vi "Interpolation.vi"() -> (2 "Flywheel Interp":dbl, 3 "Hood Interp":dbl format="%0.2f")   [LabVIEW 2025]
uses:
  <vilib>/Rock Robotics/Network Tables/NT Read Number.vi
  Framework/Robot Global Data.vi
  <vilib>/gmath/NI_Gmath.lvlib
  <vilib>/ptbypt/NI_PtbyPt.lvlib
panel:
  out "Distance to hub":dbl
  in  "Flywheel Long":dbl[](array[numeric])=[0.0, 2000.0, 2000.0, 2500.0, 2500.0, 2500.0, 2500.0, 2500.0, 2500.0, 2500.0, 3000.0, 3000.0, 3500.0, 3500.0]
  in  "Hood Long":dbl[](array[numeric])=[0.0, 40.0, 35.0, 32.0, 30.0, 25.0, 22.0, 19.0, 16.0, 13.0, 10.0, 8.0, 4.5, 2.5]
  in  "Distances Long":dbl[](array[numeric])=[0.0, 63.207, 78.8079, 85.5428, 94.7436, 106.213, 113.25, 133.336, 150.843, 165.063, 172.918, 195.81, 222.008, 256.275]
  in  "Flywheel":dbl[](array[numeric])=[3200.0, 3400.0, 3650.0, 3750.0, 3850.0, 4050.0, 4150.0, 4500.0, 4900.0, 2500.0, 3000.0, 3000.0, 3500.0, 3500.0]
  in  "Hood":dbl[](array[numeric])=[2850.0, 2900.0, 3100.0, 3200.0, 3250.0, 3350.0, 3400.0, 3900.0, 4200.0, 13.0, 10.0, 8.0, 4.5, 2.5]
  in  "Distances":dbl[](array[numeric])=[4.35402, 5.41468, 6.21537, 7.05234, 7.9447, 8.90908, 9.99438, 10.7736, 11.912, 165.063, 172.918, 195.81, 222.008, 256.275]
  # "last is unknown"
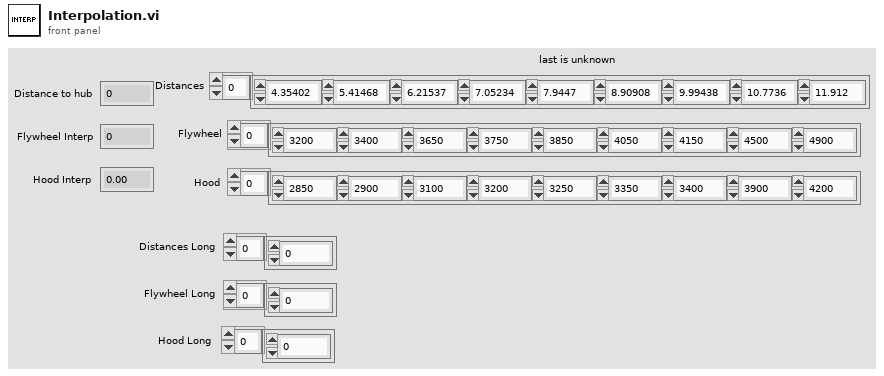
[diagram p1: front panel]
types:
  T1 = typedef "Robot Velocities.ctl" = cluster{"X Velocity":dbl, "Y Velocity":dbl, "Rotational \nVelocity":dbl}
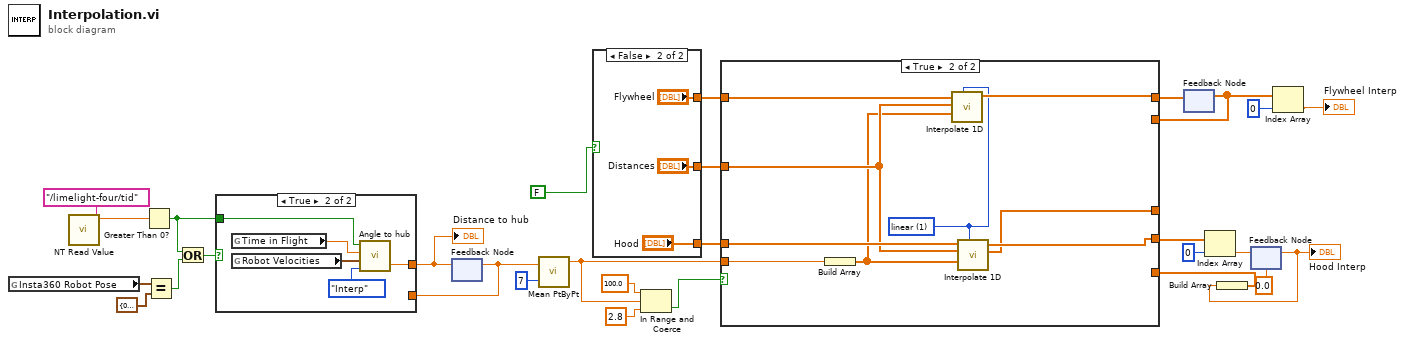
[diagram p0: block diagram]
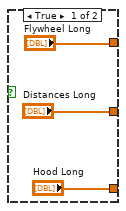
[diagram p3: hidden frame]
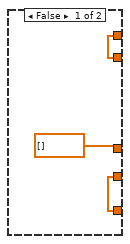
[diagram p4: hidden frame]
diagram:
  n1 = global read "Robot Global Data.vi" "Insta360 Robot Pose"() -> (w3:cluster{"X":dbl, "Y":dbl})
  n2 = call-poly <vilib>:"NT Read Value.vi"("name"="/limelight-four/tid") -> ("value"=w10:dbl)  [unwired: 8 in, 2 out]
  n3 = Greater Than 0?(x=w10) -> (x > 0?=w4:bool)
  n4 = Equal?(x=w3, y=cluster{"X":dbl, "Y":dbl} {"X"=0.0, "Y"=0.0}) -> (x = y?=w1:bool)
  n5 = Or(x=w4, y=w1) -> (x .or. y?=w5:bool)
  n6 = feedback #1() -> (w8:dbl)  [unwired: 1 in]
  n7 = case shown="True" w5 {
    tunnel: [w29 w34] -> w6
    tunnel: w8 -> [w29 _]
    tunnel: w4 -> [_ w30]
    frame False {
    }
    frame True {
      n8 = global read "Robot Global Data.vi" "Time in Flight"() -> (w32:dbl)
      n9 = global read "Robot Global Data.vi" "Robot Velocities"() -> (w31:T1)
      n10 = call "Angle to hub.vi"("Calculation Mode"=enum16{"Theta Align", "Interp"}."Interp", "Robot Velocities In"=w31, "Time in flight"=w32, "Using Limelight?"=w30) -> ("Distance to hub"=w34:dbl)  [unwired: 1 out]
    }
  }
  "Distance to hub" <- w6
  n11 = feedback-in #1(w6) -> ()
  n12 = call <vilib>:"Mean PtByPt.vi"("x"=w8, "sample length"=7) -> ("mean"=w7:dbl)  [unwired: 2 in, 1 out]
  n13 = case shown="False" FALSE {
    tunnel: ["Flywheel Long" "Flywheel"] -> w28
    tunnel: ["Hood Long" "Hood"] -> w25
    tunnel: ["Distances Long" "Distances"] -> w24
    frame True {
    }
    frame False {
    }
  }
  n14 = In Range and Coerce(upper limit=100.0, x=w7, lower limit=2.8) -> (In Range?=w14:bool)  [unwired: 1 out]
  n15 = feedback #2() -> (w18:dbl[])  [unwired: 1 in]
  n16 = feedback #3(0.0) -> (w13:dbl)
  "Hood Interp" <- w13
  n17 = Build Array(w13) -> (w15:dbl[])
  n18 = case shown="True" w14 {
    tunnel: w28 -> [_ w50]
    tunnel: [w43 w47] -> w26
    tunnel: w25 -> [_ w52]
    tunnel: [w42 w51] -> w21
    tunnel: w24 -> [_ w49]
    tunnel: w18 -> [w43 _]
    tunnel: w15 -> [w42 _]
    tunnel: [dbl[] [] ("xi used") w46] -> _
    tunnel: w7 -> [_ w45]
    frame False {
    }
    frame True {
      w44 = 1 items=["nearest", "linear", "spline", "cubic Hermite", "Lagrange"] ("method")
      n19 = Build Array(w45) -> (w48:dbl[])
      n20 = call <vilib>:"Interpolate 1D.vi"("method"=w44, "xi"=w48, "X"=w49, "Y"=w50) -> ("yi"=w47:dbl[])  [unwired: 5 in, 2 out]
      n21 = call <vilib>:"Interpolate 1D.vi"("method"=w44, "xi"=w48, "X"=w49, "Y"=w52) -> ("xi used"=w46:dbl[], "yi"=w51:dbl[])  [unwired: 5 in, 1 out]
    }
  }
  n22 = feedback-in #2(w26) -> ()
  n23 = Index Array(array=w21, index=0) -> (element=w19:dbl)
  n24 = feedback-in #3(w19) -> ()
  n25 = Index Array(array=w18, index=0) -> (element=→"Flywheel Interp":dbl)
